vi "CheckPath.vi"(0 "Path":path, 5 "error in (no error)":errorcluster) -> (14 "Restart required":bool, 19 "error out":errorcluster)   [LabVIEW 2019, in "LcWebView.lvclass"]
doc: "Check if the data folder containing required dlls to be installed in PATH variable"
uses:
  LcWebView.lvclass
  <vilib>/registry/registry.llb/Registry RtKey.ctl
  Program Files/National Instruments/LabVIEW 2020/user.lib/_OpenG.lib/array/array.llb/Remove Duplicates from 1D Array (String)__ogtk.vi
  <vilib>/registry/registry.llb/Write Registry Value Simple STR.vi
  <vilib>/registry/registry.llb/Registry SAM.ctl
  <vilib>/registry/registry.llb/Read Registry Value Simple STR.vi
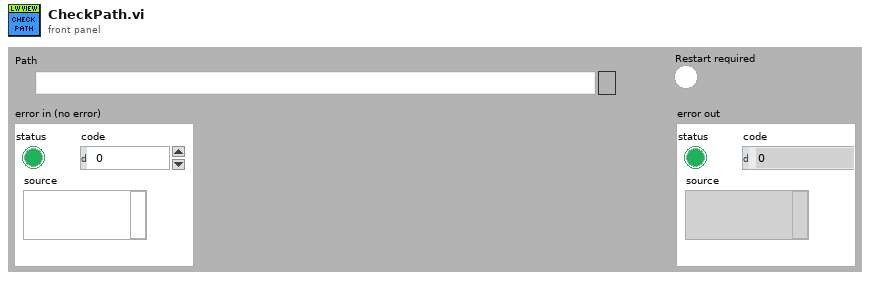
[diagram p1: front panel]
types:
  T1 = typedef "Registry SAM.ctl" = enum32{"KEY_QUERY_VALUE", "KEY_SET_VALUE", "KEY_CREATE_SUB_KEY", "KEY_ENUMERATE_SUB_KEYS", "KEY_NOTIFY", "KEY_CREATE_LINK", "KEY_READ", "KEY_WRITE", "KEY_ALL_ACCESS", "KEY_READ | KEY_WRITE"}
  T2 = typedef "Registry RtKey.ctl" = enum32{"HKEY_CLASSES_ROOT", "HKEY_CURRENT_USER", "HKEY_LOCAL_MACHINE", "HKEY_USERS", "HKEY_PERFORMANCE_DATA", "HKEY_CURRENT_CONFIG", "HKEY_DYN_DATA"}
  T3 = typedef "Registry refnum.ctl" = refnum<k1>
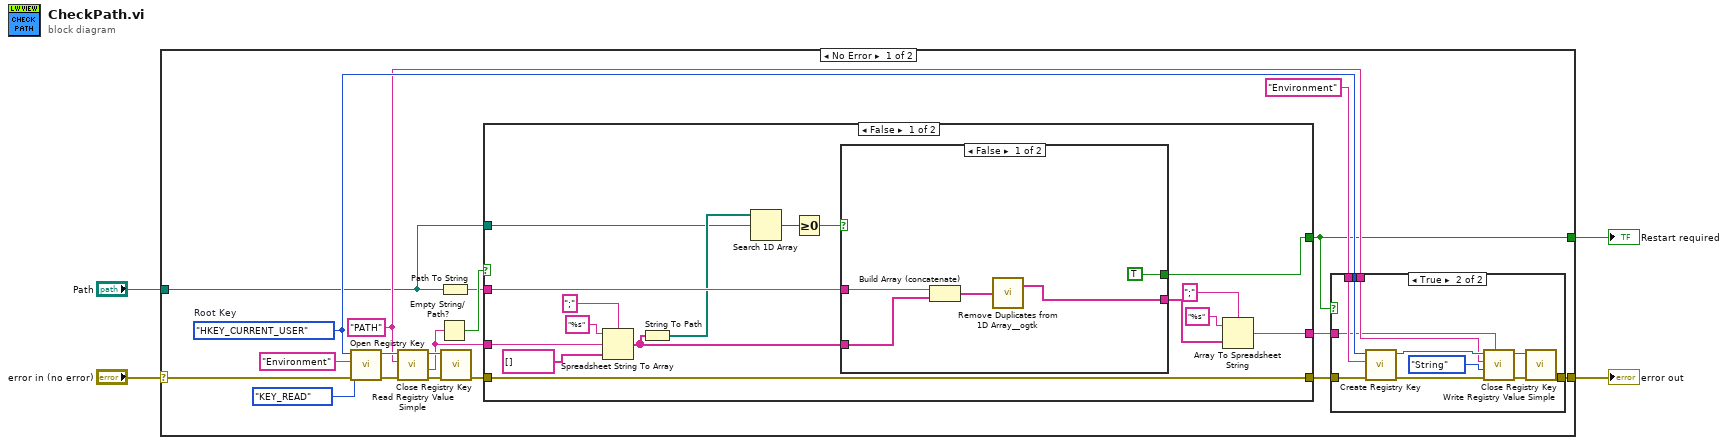
[diagram p0: block diagram]
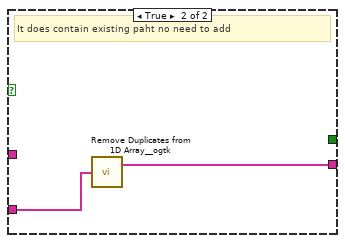
[diagram p3: hidden frame]
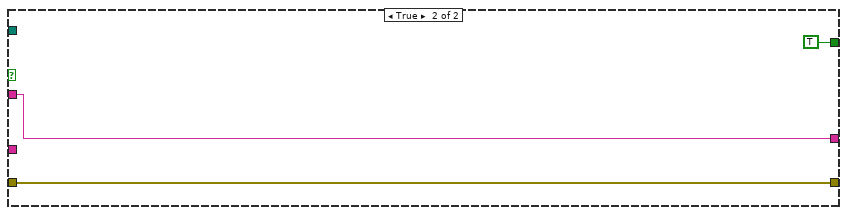
[diagram p4: hidden frame]
diagram:
  n1 = case shown="No Error" "error in (no error)" {
    selector: "error in (no error)" -> [w20 w62]
    tunnel: [w14 w62] -> w3
    tunnel: "Path" -> [w5 _]
    tunnel: [w7 _] -> w1
    frame No Error {
      w10 = "PATH" ("value")
      w13 = Registry_RtKey."HKEY_CURRENT_USER"  # Root Key
      n2 = call <vilib>:"Open Registry Key.vi"("error in (no error)"=w20, "security access mask (KEY_READ | KEY_WRITE)"=Registry_SAM."KEY_READ", "subkey"="Environment", "root key (HKEY_LOCAL_MACHINE)"=w13) -> ("error out"=w21:errorcluster, "refnum out"=w22:T3)  [unwired: 6 in]
      n3 = call-poly <vilib>:"Read Registry Value Simple.vi"("error in (no error)"=w21, "value"=w10, "refnum"=w22) -> ("error out"=w18:errorcluster, "String/Binary data"=w8:string, "refnum out"=w17:T3)  [unwired: 3 in, 1 out]
      n4 = Empty String/Path?(string/path=w8) -> (empty?=w19:bool)
      n5 = Path To String(path=w5) -> (string=w11:string)
      n6 = call <vilib>:"Close Registry Key.vi"("error in (no error)"=w18, "refnum"=w17) -> ("error out"=w16:errorcluster)  [unwired: 5 in]
      n7 = case shown="False" w19 {
        tunnel: w16 -> [w51 w61]
        tunnel: [w51 w61] -> w15
        tunnel: w11 -> [w46 w60]
        tunnel: [w41 w60] -> w9
        tunnel: w8 -> [w49 _]
        tunnel: [w45 TRUE] -> w7
        tunnel: w5 -> [w36 _]
        frame False {
          n8 = Spreadsheet String To Array(delimiter (Tab)=";", format string="%s", spreadsheet string=w49, array type (2D Dbl)=string[] [] ("format string")) -> (array=w40:string[])
          n9 = String To Path(string=w40) -> (path=w37:path[])
          n10 = Search 1D Array(1D array=w37, element=w36) -> (index of element=w39:i32)  [unwired: 1 in]
          n11 = Greater Or Equal To 0?(x=w39) -> (x >= 0?=w38:bool)
          n12 = case shown="False" w38 {
            tunnel: w46 -> [w56 _]
            tunnel: [TRUE _] -> w45
            tunnel: [w54 w57] -> w44
            tunnel: w40 -> [w53 w58]
            frame False {
              n13 = Build Array (concatenate)(w56, w53) -> (w52:string[])
              n14 = call-poly "Remove Duplicates from 1D Array__ogtk.vi"("Input Array"=w52) -> ("Output Array"=w54:string[])  [unwired: 1 out]
            }
            frame True {
              # "It does contain existing paht no need to add"
              n15 = call-poly "Remove Duplicates from 1D Array__ogtk.vi"("Input Array"=w58) -> ("Output Array"=w57:string[])  [unwired: 1 out]
            }
          }
          n16 = Array To Spreadsheet String(delimiter (Tab)=";", array=w44, 3:"%s" ("format string")) -> (spreadsheet string=w41:string)
        }
        frame True {
        }
      }
      n17 = case shown="True" w7 {
        tunnel: w15 -> [w24 w35]
        tunnel: [w24 w32] -> w14
        tunnel: w13 -> [_ w29]
        tunnel: "Environment" ("subkey") -> [_ w28]
        tunnel: w10 -> [_ w26]
        tunnel: w9 -> [_ w25]
        frame False {
        }
        frame True {
          n18 = call <vilib>:"Create Registry Key.vi"("error in (no error)"=w35, "subkey"=w28, "root key (HKEY_LOCAL_MACHINE)"=w29) -> ("error out"=w34:errorcluster, "refnum out"=w31:T3)  [unwired: 6 in, 1 out]
          n19 = call-poly <vilib>:"Write Registry Value Simple.vi"("String/Binary data"=w25, "error in (no error)"=w34, "simple data type"=enum16{"String", "Binary", "DWORD"}."String", "value"=w26, "refnum"=w31) -> ("error out"=w33:errorcluster, "refnum out"=w30:T3)  [unwired: 3 in]
          n20 = call <vilib>:"Close Registry Key.vi"("error in (no error)"=w33, "refnum"=w30) -> ("error out"=w32:errorcluster)  [unwired: 5 in]
        }
      }
    }
    frame Error {
    }
  }
  "error out" <- w3
  "Restart required" <- w1
